vi "Command Drive Distance Ramp.vi"(8 "Ramp_Distance":dbl=42.0, 9 "Heading":dbl=50.0, 10 "Distance":dbl=42.0, 11 "Startup":bool) -> (0 "Right Wheel":dbl, 1 "Reinit":bool, 2 "Left Wheel":dbl, 3 "Completed":bool=TRUE)   [LabVIEW 2017]
uses:
  Utility VIs/Refnum Names.vi
  Drive/Drive Globals.vi
panel:
  in  "Turn Gain":dbl=0.06
  in  "Gain":dbl=0.028
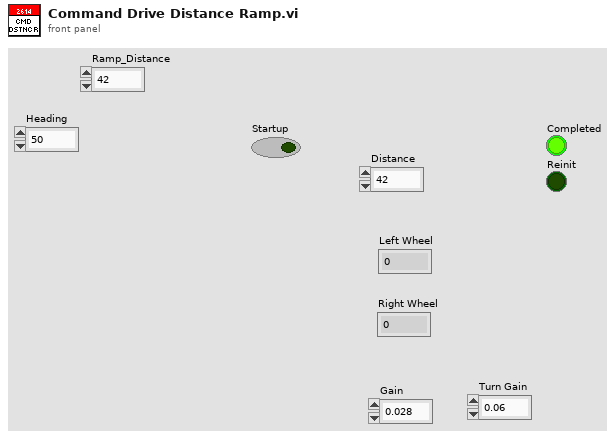
[diagram p1: front panel]
types:
  T1 = typedef "WPI_MotorControlDeviceRef.ctl" = cluster{"DeviceStatus":errorcluster, "Type":T2, "PWM":cluster{"PWM Channel":T3, "DeadBand":T4}, "CAN":cluster{"Device Number":u8, "SetOutput VI Ref":variant, "GetOutput VI Ref":variant, "Enable VI Ref":variant, "Disable VI Ref":variant, "Data":variant}, "Invert":bool, "DIO PWM":cluster{"PWM \"Enable\" Channel":T3, "DIOChannel":T5, "PWM Rate":dbl}}
  T2 = typedef "WPI_MotorControlType.ctl" = enum16{"PWM", "CAN", "DIO PWM"}
  T3 = typedef "FPGA_DIOPWMChannel.ctl" = enum8{"PWM 0", "PWM 1", "PWM 2", "PWM 3", "PWM 4", "PWM 5", "PWM 6", "PWM 7", "PWM 8", "PWM 9", "PWM MXP 0", "PWM MXP 1", "PWM MXP 2", "PWM MXP 3", "PWM MXP 4", "PWM MXP 5", "PWM MXP 6", "PWM MXP 7", "PWM MXP 8", "PWM MXP 9", "Invalid"}
  T4 = typedef "WPI_PWMDeadband.ctl" = cluster{"Name":string, "maxPositivePwm":i32, "minPositivePwm":i32, "centerPwm":i32, "maxNegativePwm":i32, "minNegativePwm":i32, "angularRange":u16}
  T5 = typedef "FPGA_DIOChannel.ctl" = enum8{"DIO 0", "DIO 1", "DIO 2", "DIO 3", "DIO 4", "DIO 5", "DIO 6", "DIO 7", "DIO 8", "DIO 9", "DIO MXP 0", "DIO MXP 1", "DIO MXP 2", "DIO MXP 3", "DIO MXP 4", "DIO MXP 5", "DIO MXP 6", "DIO MXP 7", "DIO MXP 8", "DIO MXP 9", "DIO MXP 10", "DIO MXP 11", "DIO MXP 12", "DIO MXP 13", "DIO MXP 14", "DIO MXP 15", "SPI Port CS1", "SPI Port CS2", "SPI Port CS3", "SPI Port MISO", "SPI Port MOSI", "Invalid"}
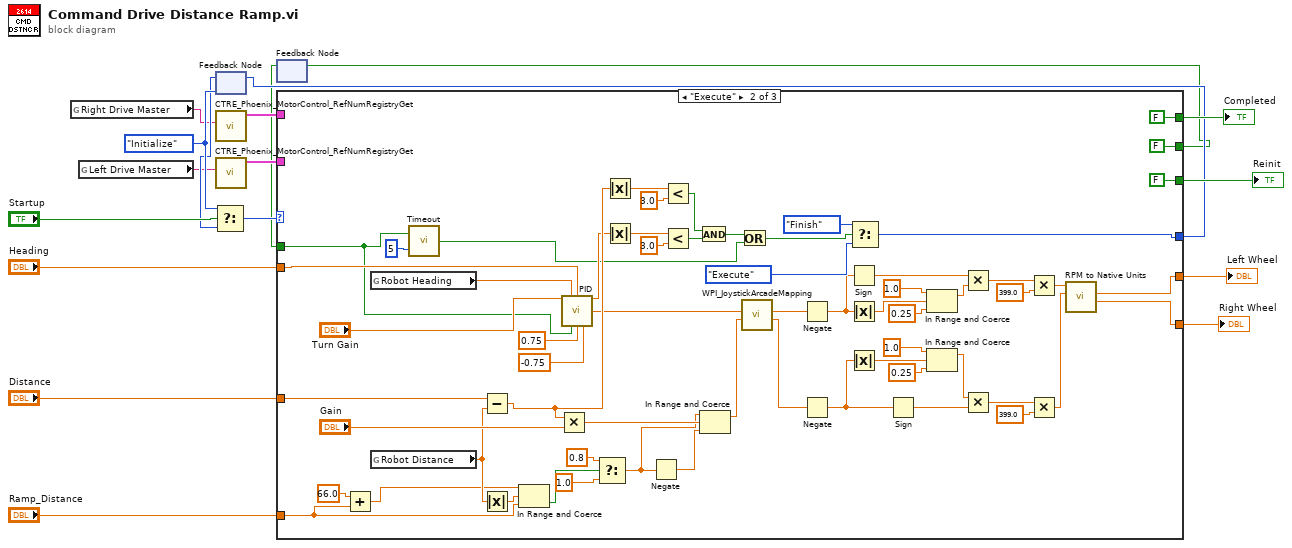
[diagram p0: block diagram]
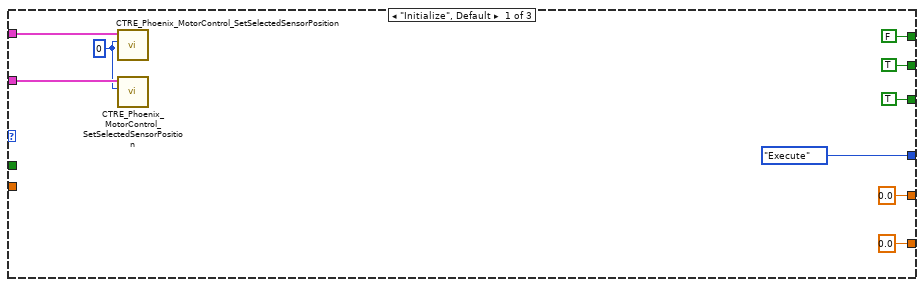
[diagram p2: hidden frame]
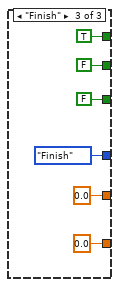
[diagram p3: hidden frame]
diagram:
  w16 = enum16{"Initialize", "Execute", "Finish"}."Initialize"
  n1 = global read "Refnum Names.vi" "Right Drive Master"() -> (w7:string)
  n2 = global read "Refnum Names.vi" "Left Drive Master"() -> (w8:string)
  n3 = feedback #1(w16) -> (w12:enum16{"Initialize", "Execute", "Finish"})
  n4 = Select(t=w16, s="Startup", f=w12) -> (s? t:f=w17:enum16{"Initialize", "Execute", "Finish"})
  n5 = call <vilib>:"CTRE_Phoenix_MotorControl_RefNumRegistryGet.vi"("refnum name"=w7) -> ("PhoenixMotorControlDevRef"=w6:T1)  [unwired: 9 in, 1 out]
  n6 = call <vilib>:"CTRE_Phoenix_MotorControl_RefNumRegistryGet.vi"("refnum name"=w8) -> ("PhoenixMotorControlDevRef"=w5:T1)  [unwired: 9 in, 1 out]
  n7 = feedback #2() -> (w2:bool)  [unwired: 1 in]
  n8 = case shown="\"Execute\"" w17 {
    tunnel: [FALSE FALSE TRUE] -> w15
    tunnel: [TRUE FALSE FALSE] -> w14
    tunnel: [enum16{"Initialize", "Execute", "Finish"}."Execute" w85 enum16{"Initialize", "Execute", "Finish"}."Finish"] -> w13
    tunnel: "Distance" -> [_ w84 _]
    tunnel: [0.0 ("Left Wheel Velocity") w41 0.0] -> w10
    tunnel: [0.0 ("Right Wheel Velocity") w40 0.0] -> w9
    tunnel: w6 -> [w21 _ _]
    tunnel: w5 -> [w22 _ _]
    tunnel: "Heading" -> [_ w67 _]
    tunnel: [TRUE FALSE FALSE] -> w3
    tunnel: w2 -> [_ w28 _]
    tunnel: "Ramp_Distance" -> [_ w34 _]
    frame "Initialize", Default {
      w20 = 0
      n9 = call <vilib>:"CTRE_Phoenix_MotorControl_SetSelectedSensorPosition.vi"("New Sensor Position"=w20, "PhoenixMotorControlDevRef"=w21) -> ()  [unwired: 8 in, 2 out]
      n10 = call <vilib>:"CTRE_Phoenix_MotorControl_SetSelectedSensorPosition.vi"("New Sensor Position"=w20, "PhoenixMotorControlDevRef"=w22) -> ()  [unwired: 8 in, 2 out]
    }
    frame "Execute" {
      n11 = Add(x=66.0, y=w34) -> (x+y=w35:dbl)
      n12 = global read "Drive Globals.vi" "Robot Heading"() -> (w79:dbl)
      n13 = global read "Drive Globals.vi" "Robot Distance"() -> (w38:dbl)
      n14 = call "Timeout.vi"("Timeout"=u32 5, "Initialize"=w28) -> ("Timed Out?"=w58:bool)
      n15 = Subtract(x=w84, y=w38) -> (x-y=w81:dbl)
      n16 = Absolute Value(x=w38) -> (abs(x)=w37:dbl)
      n17 = In Range and Coerce(upper limit=w35, x=w37, lower limit=w34) -> (In Range?=w39:bool)  [unwired: 1 out]
      n18 = Multiply(x=w81, y="Gain") -> (x*y=w77:dbl)
      n19 = call "PID.vi"("Kp"="Turn Gain", "Process Variable"=w79, "Goal"=w67, "Reinit"=w28, "Max Ouput"=0.75, "Min Output"=-0.75) -> ("Current Error"=w68:dbl, "Command"=w66:dbl)  [unwired: 7 in, 1 out]
      n20 = Select(t=0.8, s=w39, f=1.0) -> (s? t:f=w30:dbl)
      n21 = Absolute Value(x=w81) -> (abs(x)=w82:dbl)
      n22 = Absolute Value(x=w68) -> (abs(x)=w70:dbl)
      n23 = Negate(x=w30) -> (-x=w29:dbl)
      n24 = Less?(x=w82, y=3.0) -> (x < y?=w72:bool)
      n25 = Less?(x=w70, y=3.0) -> (x < y?=w69:bool)
      n26 = And(x=w72, y=w69) -> (x .and. y?=w73:bool)
      n27 = In Range and Coerce(upper limit=w30, x=w77, lower limit=w29) -> (coerced(x)=w65:dbl)  [unwired: 1 out]
      n28 = Or(x=w73, y=w58) -> (x .or. y?=w59:bool)
      n29 = call <vilib>:"WPI_JoystickArcadeMapping.vi"("Y axis value"=w65, "X axis value"=w66) -> ("Right Motor Value"=w63:dbl, "Left Motor Value"=w64:dbl)  [unwired: 8 in]
      n30 = Negate(x=w64) -> (-x=w54:dbl)
      n31 = Negate(x=w63) -> (-x=w55:dbl)
      n32 = Sign(1:w54) -> (0:w53:dbl)
      n33 = Absolute Value(x=w54) -> (abs(x)=w57:dbl)
      n34 = Absolute Value(x=w55) -> (abs(x)=w56:dbl)
      n35 = Select(t=enum16{"Initialize", "Execute", "Finish"}."Finish", s=w59, f=enum16{"Initialize", "Execute", "Finish"}."Execute") -> (s? t:f=w85:enum16{"Initialize", "Execute", "Finish"})
      n36 = Sign(1:w55) -> (0:w48:dbl)
      n37 = In Range and Coerce(upper limit=1.0, x=w57, lower limit=0.25) -> (coerced(x)=w52:dbl)  [unwired: 1 out]
      n38 = In Range and Coerce(upper limit=1.0, x=w56, lower limit=0.25) -> (coerced(x)=w49:dbl)  [unwired: 1 out]
      n39 = Multiply(x=w53, y=w52) -> (x*y=w51:dbl)
      n40 = Multiply(x=w49, y=w48) -> (x*y=w50:dbl)
      n41 = Multiply(x=w51, y=399.0) -> (x*y=w43:dbl)
      n42 = Multiply(x=w50, y=399.0) -> (x*y=w42:dbl)
      n43 = call "RPM to Native Units.vi"("Right RPM"=w42, "Left RPM"=w43) -> ("Right Out"=w40:dbl, "Left Out"=w41:dbl)  [unwired: 6 in, 1 out]
    }
    frame "Finish" {
    }
  }
  "Completed" <- w15
  "Reinit" <- w14
  "Left Wheel" <- w10
  "Right Wheel" <- w9
  n44 = feedback-in #1(w13) -> ()
  n45 = feedback-in #2(w3) -> ()
